vi "sandbox.vi"() -> ()   [LabVIEW 2019]
panel:
  out "Z":dbl
  out "Y":dbl
  out "X":dbl
  out "load":dbl
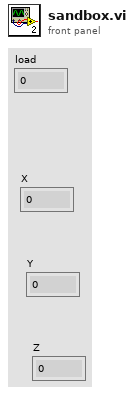
[diagram p1: front panel]
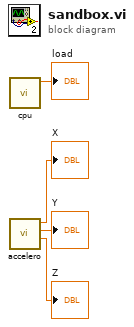
[diagram p0: block diagram]
diagram:
  n1 = call "cpu.vi"() -> ("load"=→"load":dbl)  [unwired: 11 in]
  n2 = call "accelero.vi"() -> ("Z"=→"Z":dbl, "Y"=→"Y":dbl, "X"=→"X":dbl)  [unwired: 9 in]
